vi "arm control.vi"(9 "FPGA_Time_Seconds":dbl format="%33.4f", 10 "appended array":T1[](array[typedef])) -> (2 "appended array 2":dbl[](array[numeric]))   [LabVIEW 2020]
uses:
  <vilib>/Rock Robotics/WPI/MotorControl/WPI_MotorControlDeviceRef.ctl
  <vilib>/Rock Robotics/WPI/MotorControl/WPI_MotorControlType.ctl
  <vilib>/Rock Robotics/SystemInterfaces/DIO/FPGA_DIOPWMChannel.ctl
  <vilib>/Rock Robotics/WPI/PWM/WPI_PWMDeadband.ctl
  <vilib>/Rock Robotics/SystemInterfaces/DIO/FPGA_DIOChannel.ctl
  <vilib>/Rock Robotics/WPI/Joystick/XBox Buttons Indexer.ctl
  <vilib>/Rock Robotics/WPI/Joystick/XBox Axes Indexer.ctl
  <vilib>/Rock Robotics/WPI/ThirdParty/JAS_Junk/TrajLib/PIDController_AtSetpoint.vi
  <vilib>/Rock Robotics/WPI/ThirdParty/JAS_Junk/TrajLib/PIDController_SetPIDF.vi
  <vilib>/Rock Robotics/WPI/ThirdParty/JAS_Junk/TrajLib/PIDController_SetDerivativeFilter.vi
  <vilib>/Rock Robotics/WPI/ThirdParty/JAS_Junk/TrajLib/PIDController_SetIntegratorRange.vi
  <vilib>/Rock Robotics/WPI/ThirdParty/JAS_Junk/TrajLib/PIDController_SetTolerancePandV.vi
  <vilib>/Rock Robotics/WPI/ThirdParty/JAS_Junk/TrajLib/PIDController_DisableContinousInput.vi
  <vilib>/Rock Robotics/WPI/ThirdParty/JAS_Junk/TrajLib/PIDController_EnableContinousInput.vi
  <vilib>/Rock Robotics/WPI/ThirdParty/JAS_Junk/TrajLib/PIDController_Reset.vi
  <vilib>/Rock Robotics/WPI/ThirdParty/JAS_Junk/TrajLib/PIDController_New.vi
  <vilib>/Rock Robotics/WPI/ThirdParty/JAS_Junk/TrajLib/PIDController_SetOutputLimits.vi
  <vilib>/Rock Robotics/WPI/ThirdParty/JAS_Junk/TrajLib/PIDController_NewPeriod.vi
  <vilib>/Rock Robotics/SystemInterfaces/NetworkCommunication/NetComm_UsageReport_report.vi
  Robot Global Data.vi
  <vilib>/Rock Robotics/WPI/ThirdParty/JAS_Junk/TrajLib/Globals/Util_LibraryGlobals.vi
  <vilib>/Rock Robotics/WPI/ThirdParty/JAS_Junk/TrajLib/PIDController_AdvCalculate_FF_Sp_Pv.vi
  <vilib>/Rock Robotics/WPI/ThirdParty/JAS_Junk/TrajLib/Trajectory_Library.lvlib
panel:
  in  "Kp Arm":dbl=0.33 format="%#_13g"
  out "one press\n 5":bool
  out "current angle 5":dbl
  out "current angle 3":dbl
  out "current angle 2":dbl
  out "current angle":dbl
  in  "Kd Grip":dbl format="%#_13g"
  in  "Ki Grip":dbl format="%#_13g"
  in  "Kp Grip":dbl format="%#_13g"
  in  "Kd Wirst":dbl format="%#_13g"
  in  "Ki Wrist":dbl=0.009 format="%#_13g"
  in  "Kp Wrist":dbl=0.06 format="%#_13g"
  in  "Kd Elbow":dbl format="%#_13g"
  in  "Ki Elbow":dbl=0.001 format="%#_13g"
  in  "Kp Elbow":dbl=0.04 format="%#_13g"
  in  "Kd Arm":dbl format="%#_13g"
  in  "Ki Arm":dbl=0.001 format="%#_13g"
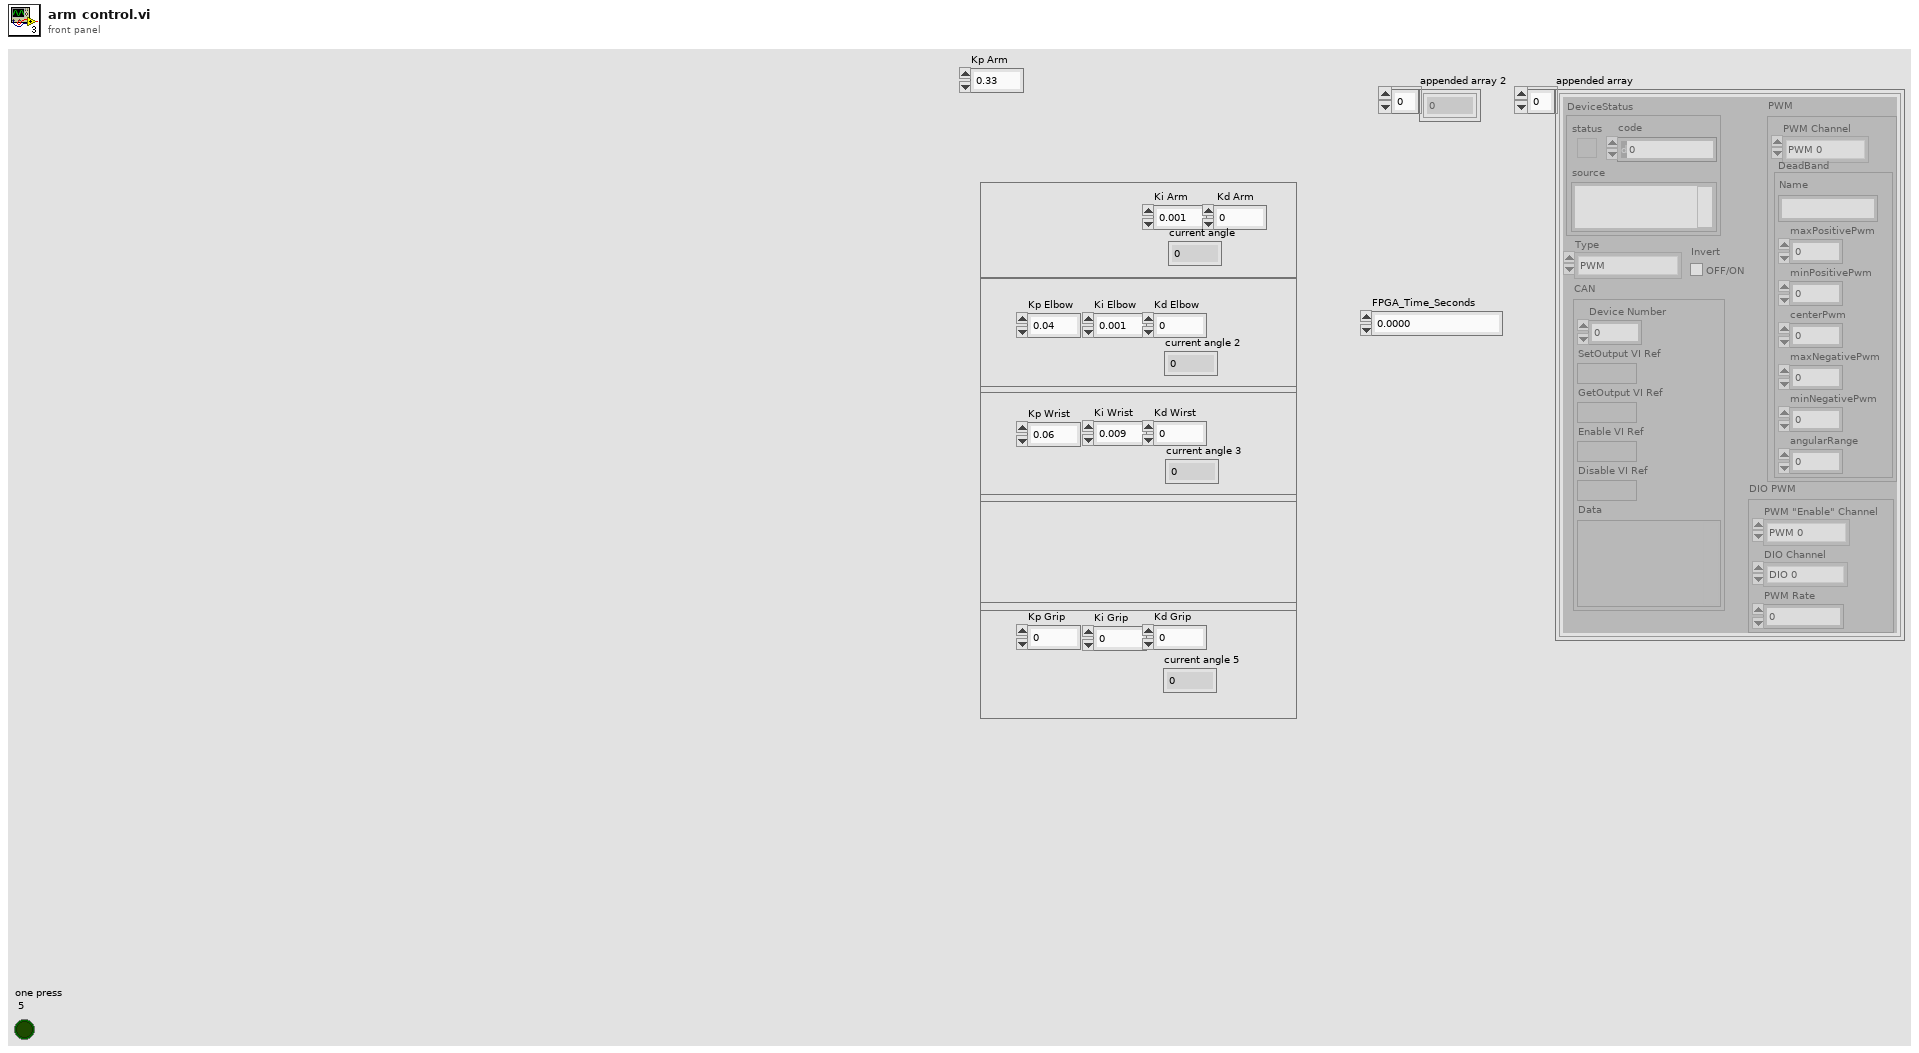
[diagram p1: front panel]
types:
  T1 = typedef "WPI_MotorControlDeviceRef.ctl" = cluster{"DeviceStatus":errorcluster, "Type":T2, "PWM":cluster{"PWM Channel":T3, "DeadBand":T4}, "CAN":cluster{"Device Number":u8, "SetOutput VI Ref":variant, "GetOutput VI Ref":variant, "Enable VI Ref":variant, "Disable VI Ref":variant, "Data":variant}, "Invert":bool, "DIO PWM":cluster{"PWM \"Enable\" Channel":T3, "DIOChannel":T5, "PWM Rate":dbl}}
  T2 = typedef "WPI_MotorControlType.ctl" = enum16{"PWM", "CAN", "DIO PWM"}
  T3 = typedef "FPGA_DIOPWMChannel.ctl" = enum8{"PWM 0", "PWM 1", "PWM 2", "PWM 3", "PWM 4", "PWM 5", "PWM 6", "PWM 7", "PWM 8", "PWM 9", "PWM MXP 0", "PWM MXP 1", "PWM MXP 2", "PWM MXP 3", "PWM MXP 4", "PWM MXP 5", "PWM MXP 6", "PWM MXP 7", "PWM MXP 8", "PWM MXP 9", "Invalid"}
  T4 = typedef "WPI_PWMDeadband.ctl" = cluster{"Name":string, "maxPositivePwm":i32, "minPositivePwm":i32, "centerPwm":i32, "maxNegativePwm":i32, "minNegativePwm":i32, "angularRange":u16}
  T5 = typedef "FPGA_DIOChannel.ctl" = enum8{"DIO 0", "DIO 1", "DIO 2", "DIO 3", "DIO 4", "DIO 5", "DIO 6", "DIO 7", "DIO 8", "DIO 9", "DIO MXP 0", "DIO MXP 1", "DIO MXP 2", "DIO MXP 3", "DIO MXP 4", "DIO MXP 5", "DIO MXP 6", "DIO MXP 7", "DIO MXP 8", "DIO MXP 9", "DIO MXP 10", "DIO MXP 11", "DIO MXP 12", "DIO MXP 13", "DIO MXP 14", "DIO MXP 15", "SPI Port CS1", "SPI Port CS2", "SPI Port CS3", "SPI Port MISO", "SPI Port MOSI", "Invalid"}
  T6 = typedef "XBox Buttons Indexer.ctl" = enum16{"A", "B", "X", "Y", "Left Bumper", "Right Bumper", "Back", "Start", "Left Joystick", "Right Joystick"}
  T7 = typedef "XBox Axes Indexer.ctl" = enum16{"Left X", "Left Y", "Left Trigger", "Right Trigger", "Right X", "Right Y"}
  T8 = typedef "Trajectory_Library.lvlib/PID_ADV_LIMITS.ctl" = cluster{"MaxInput":dbl, "MinInput":dbl, "Continuous":bool, "MaxOutput":dbl, "MinOutput":dbl}
  T9 = typedef "Trajectory_Library.lvlib/PID_ADV_TUNING.ctl" = cluster{"Kf":dbl, "Kp":dbl, "Ki":dbl, "Kd":dbl, "MaximumIntegral":dbl, "MinimumIntegral":dbl, "Filter Derivative":bool}
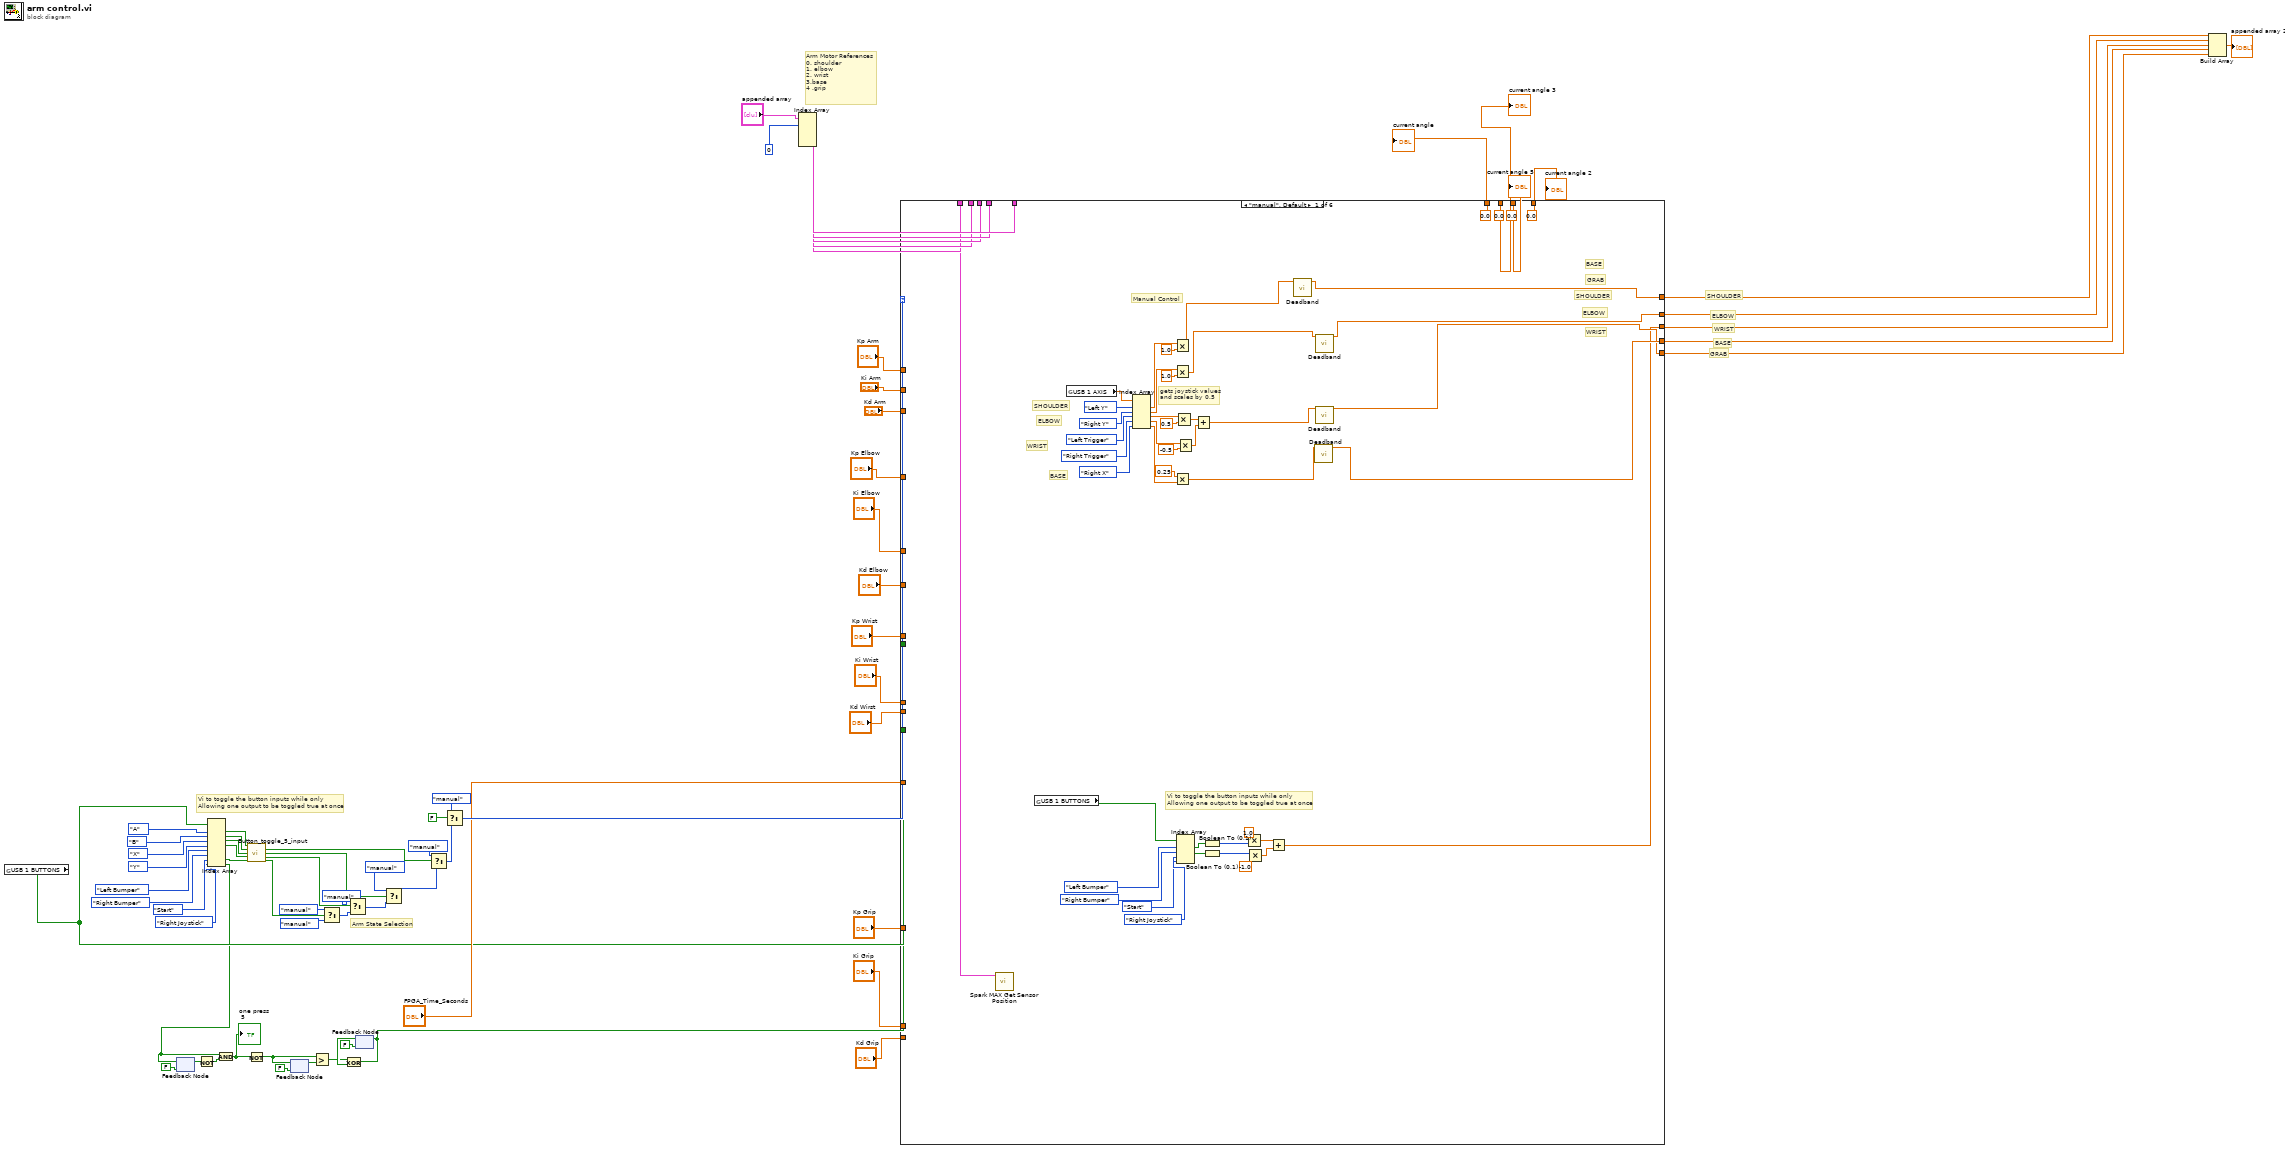
[diagram p0: block diagram]
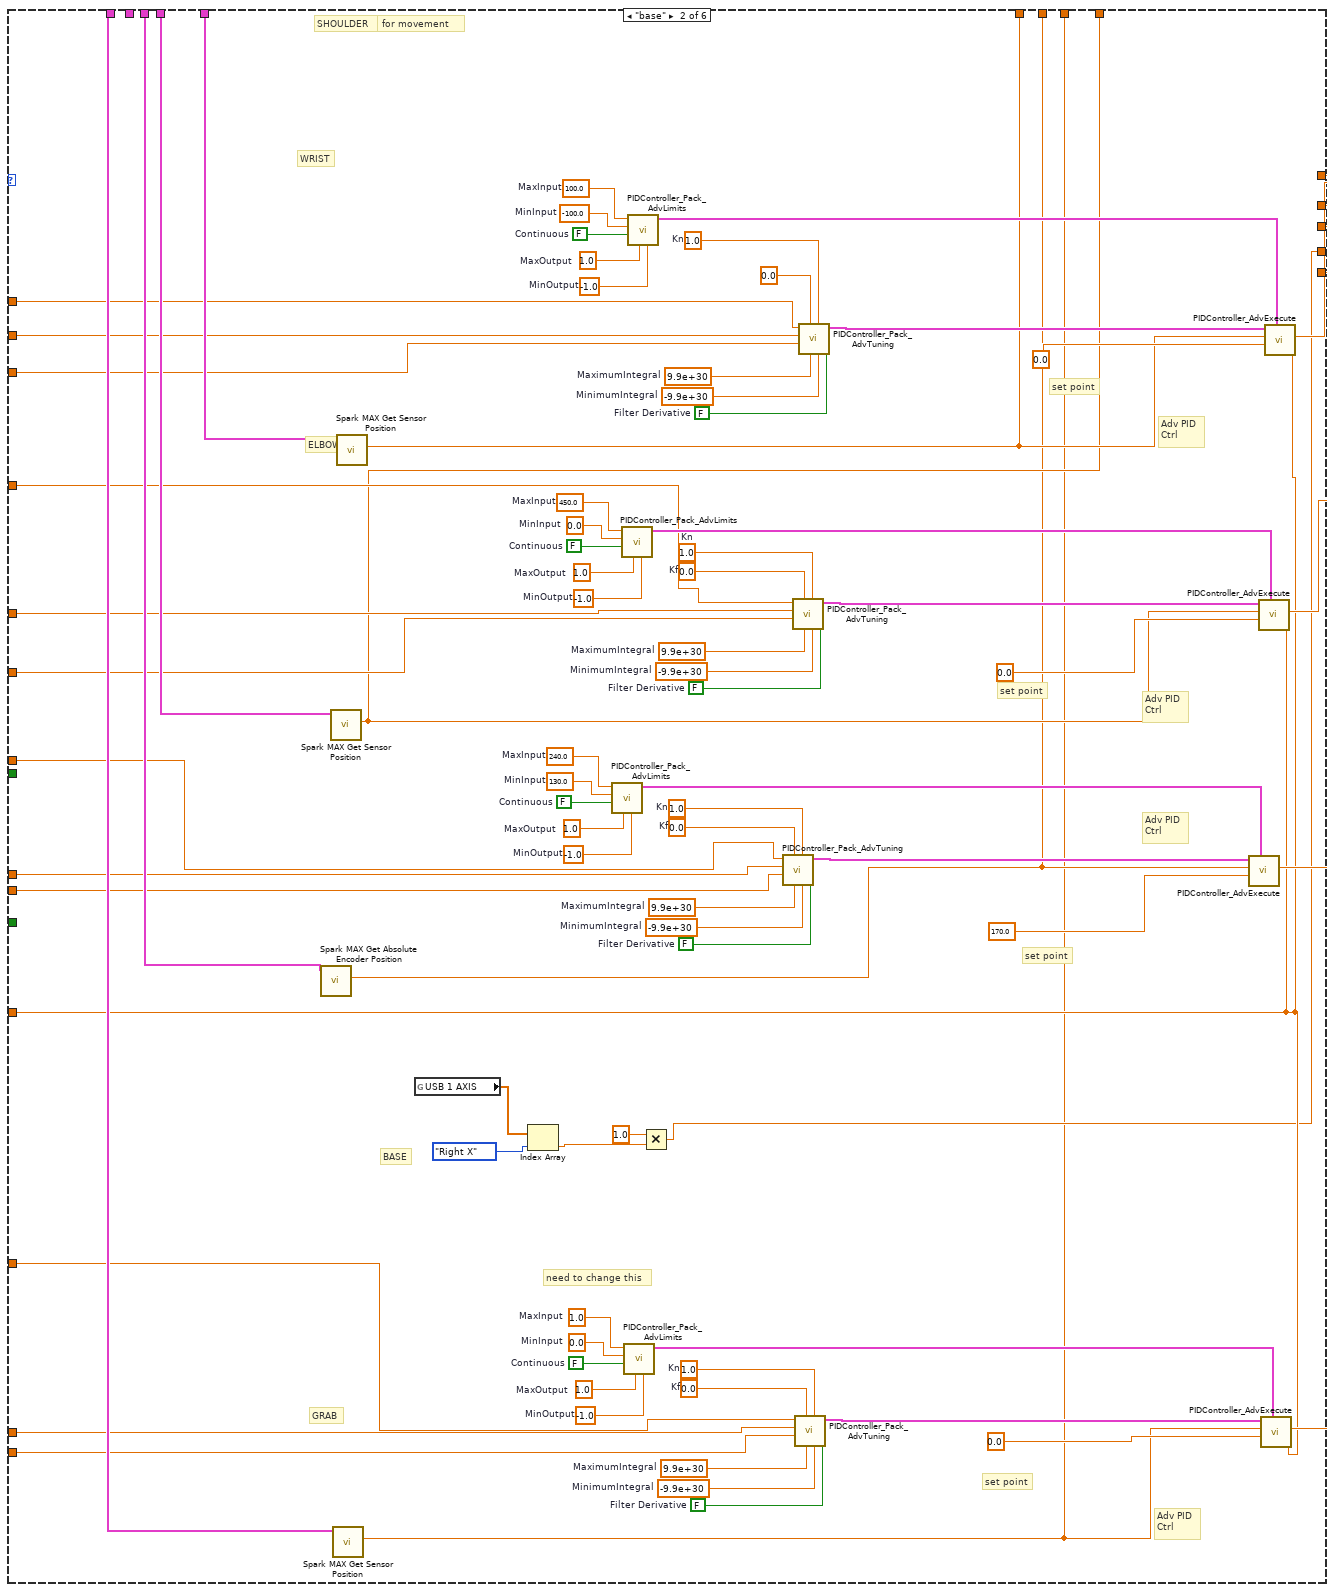
[diagram p2: hidden frame]
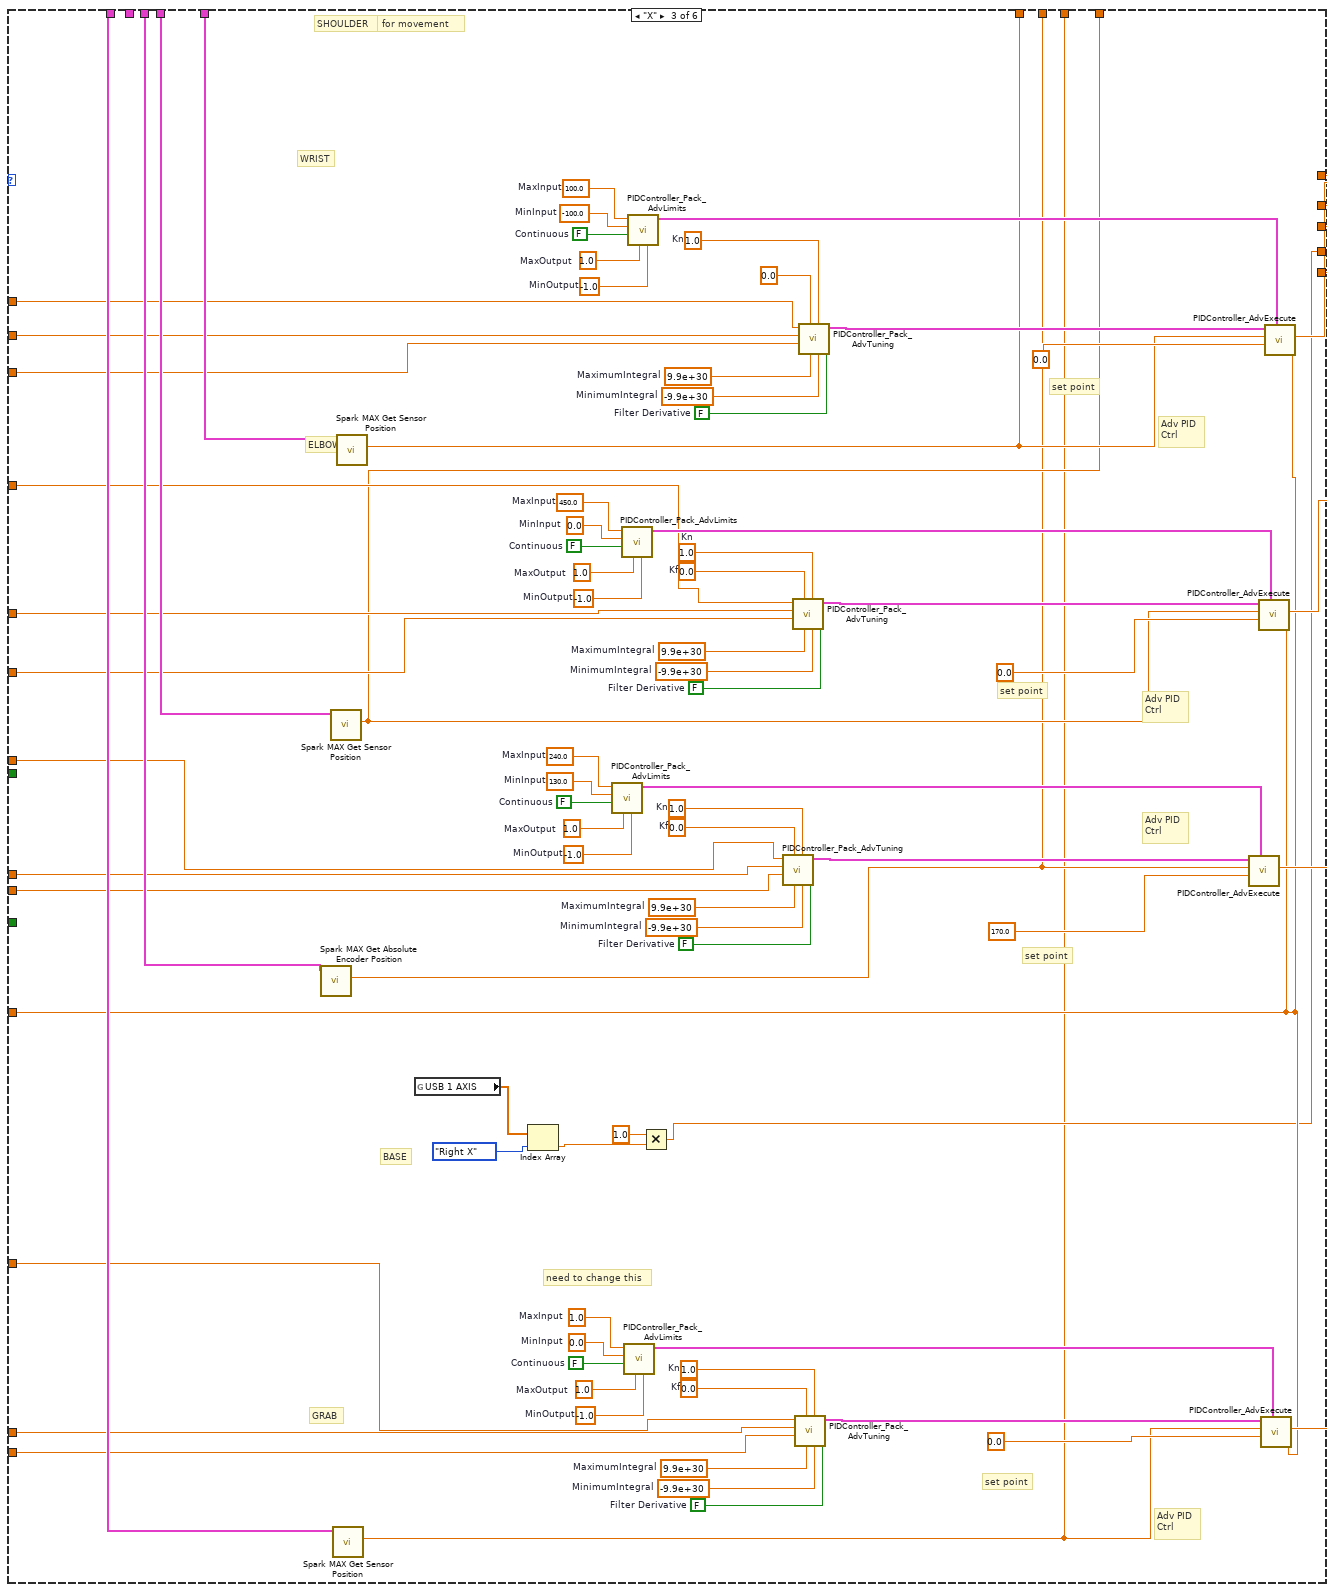
[diagram p3: hidden frame]
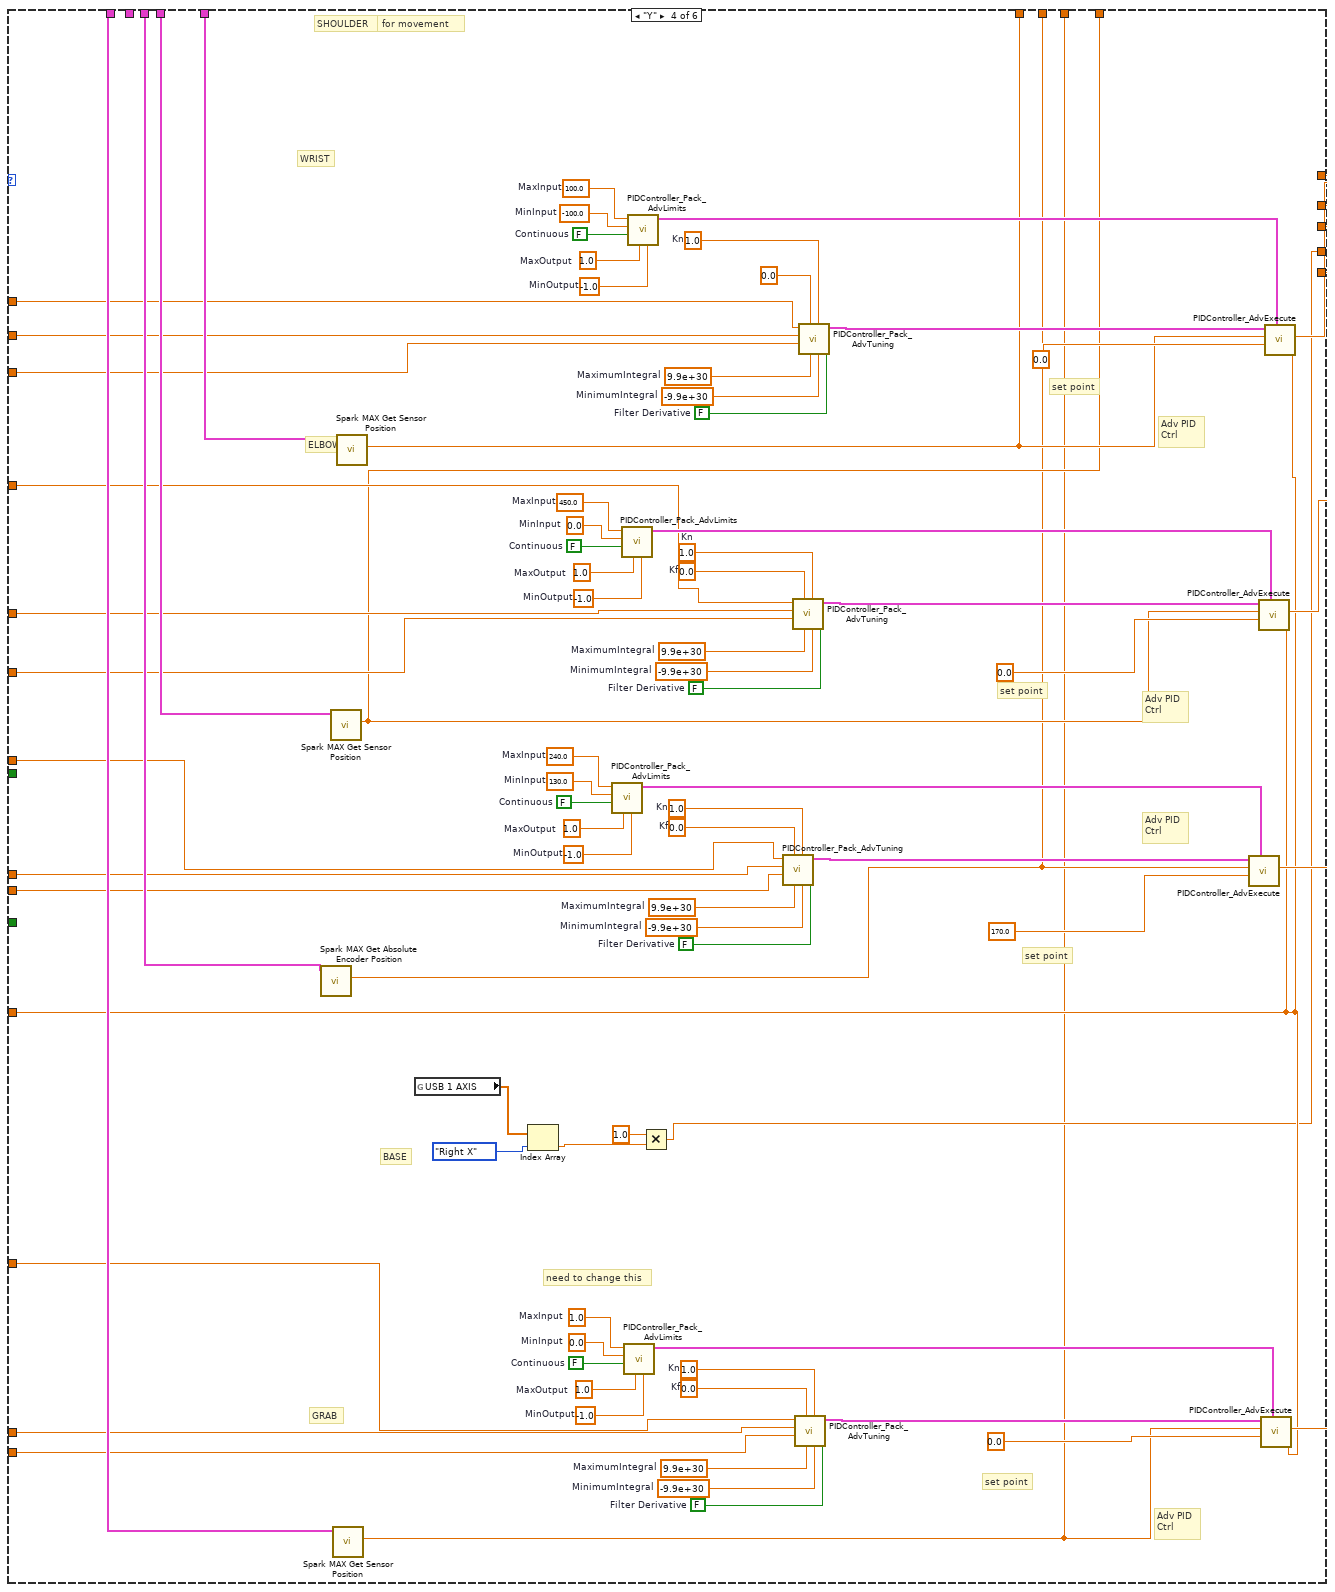
[diagram p4: hidden frame]
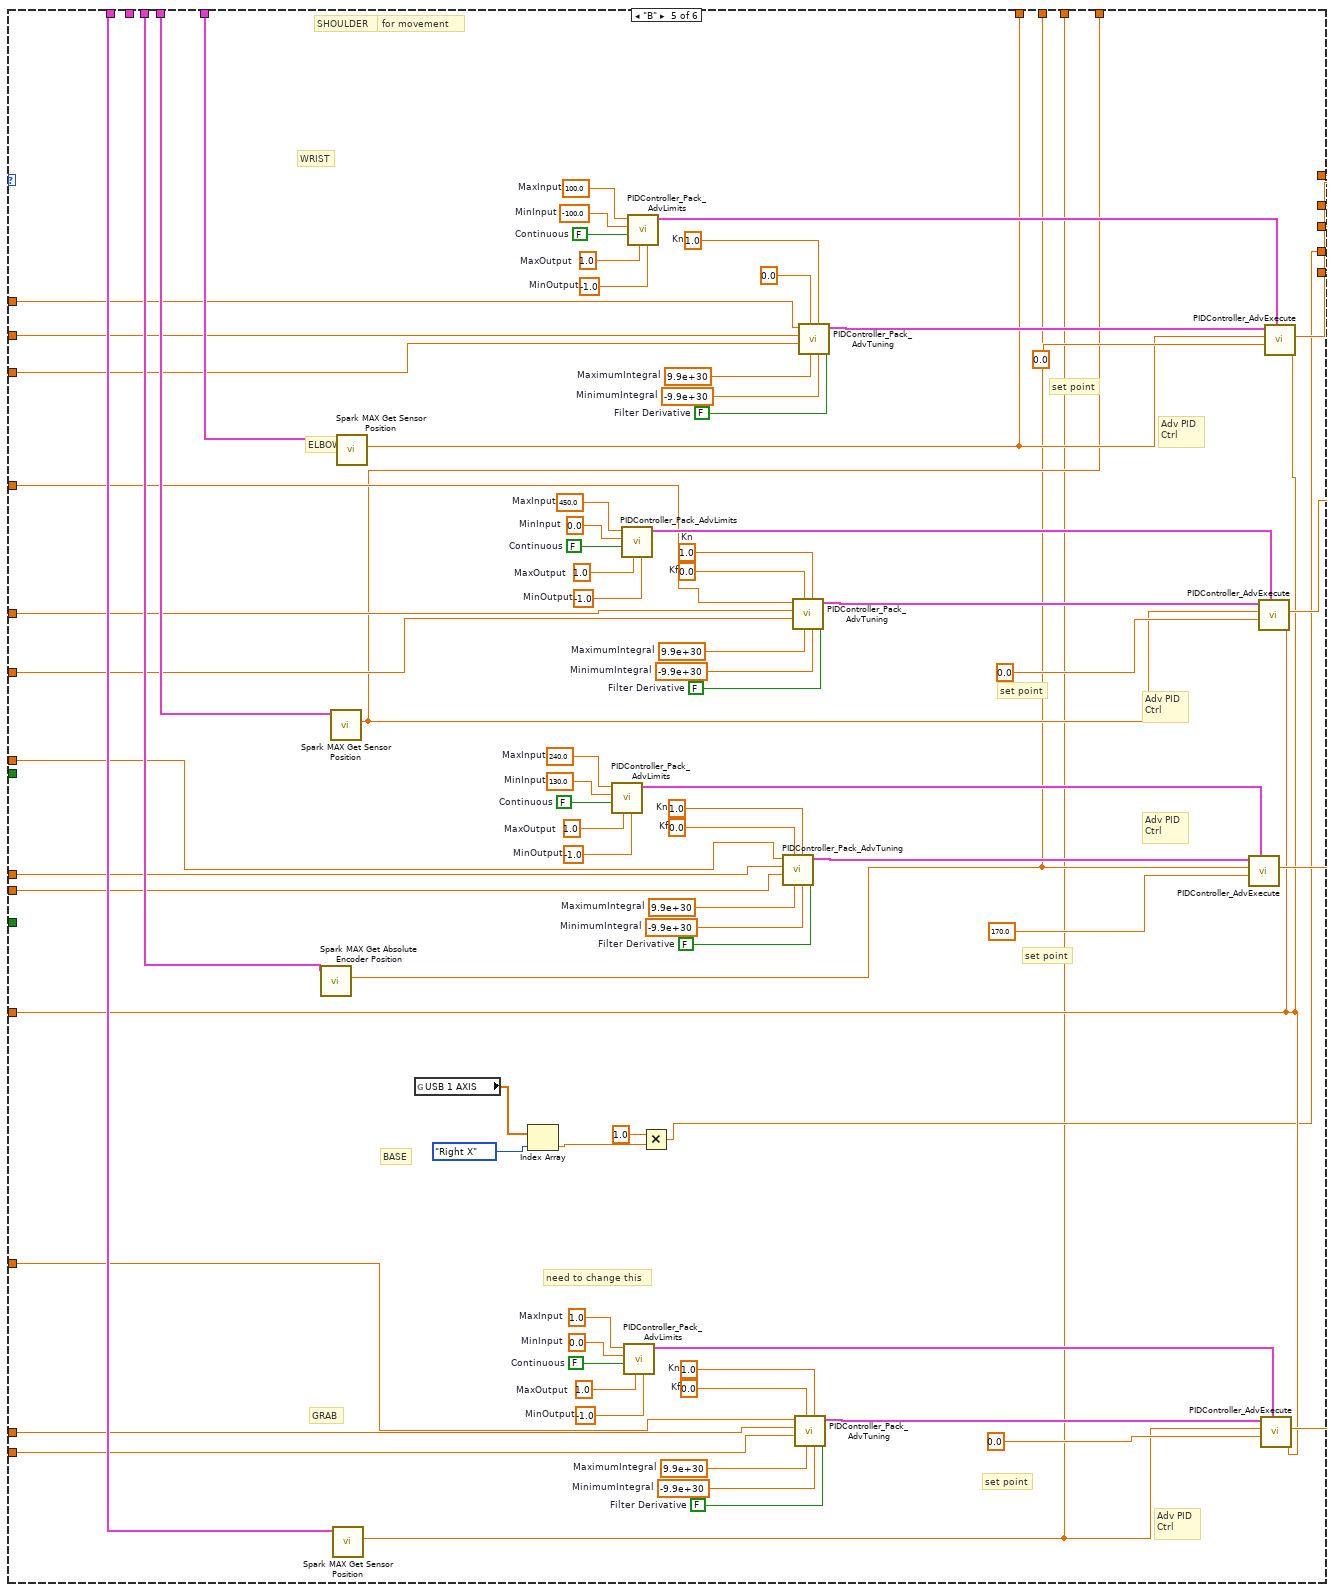
[diagram p5: hidden frame]
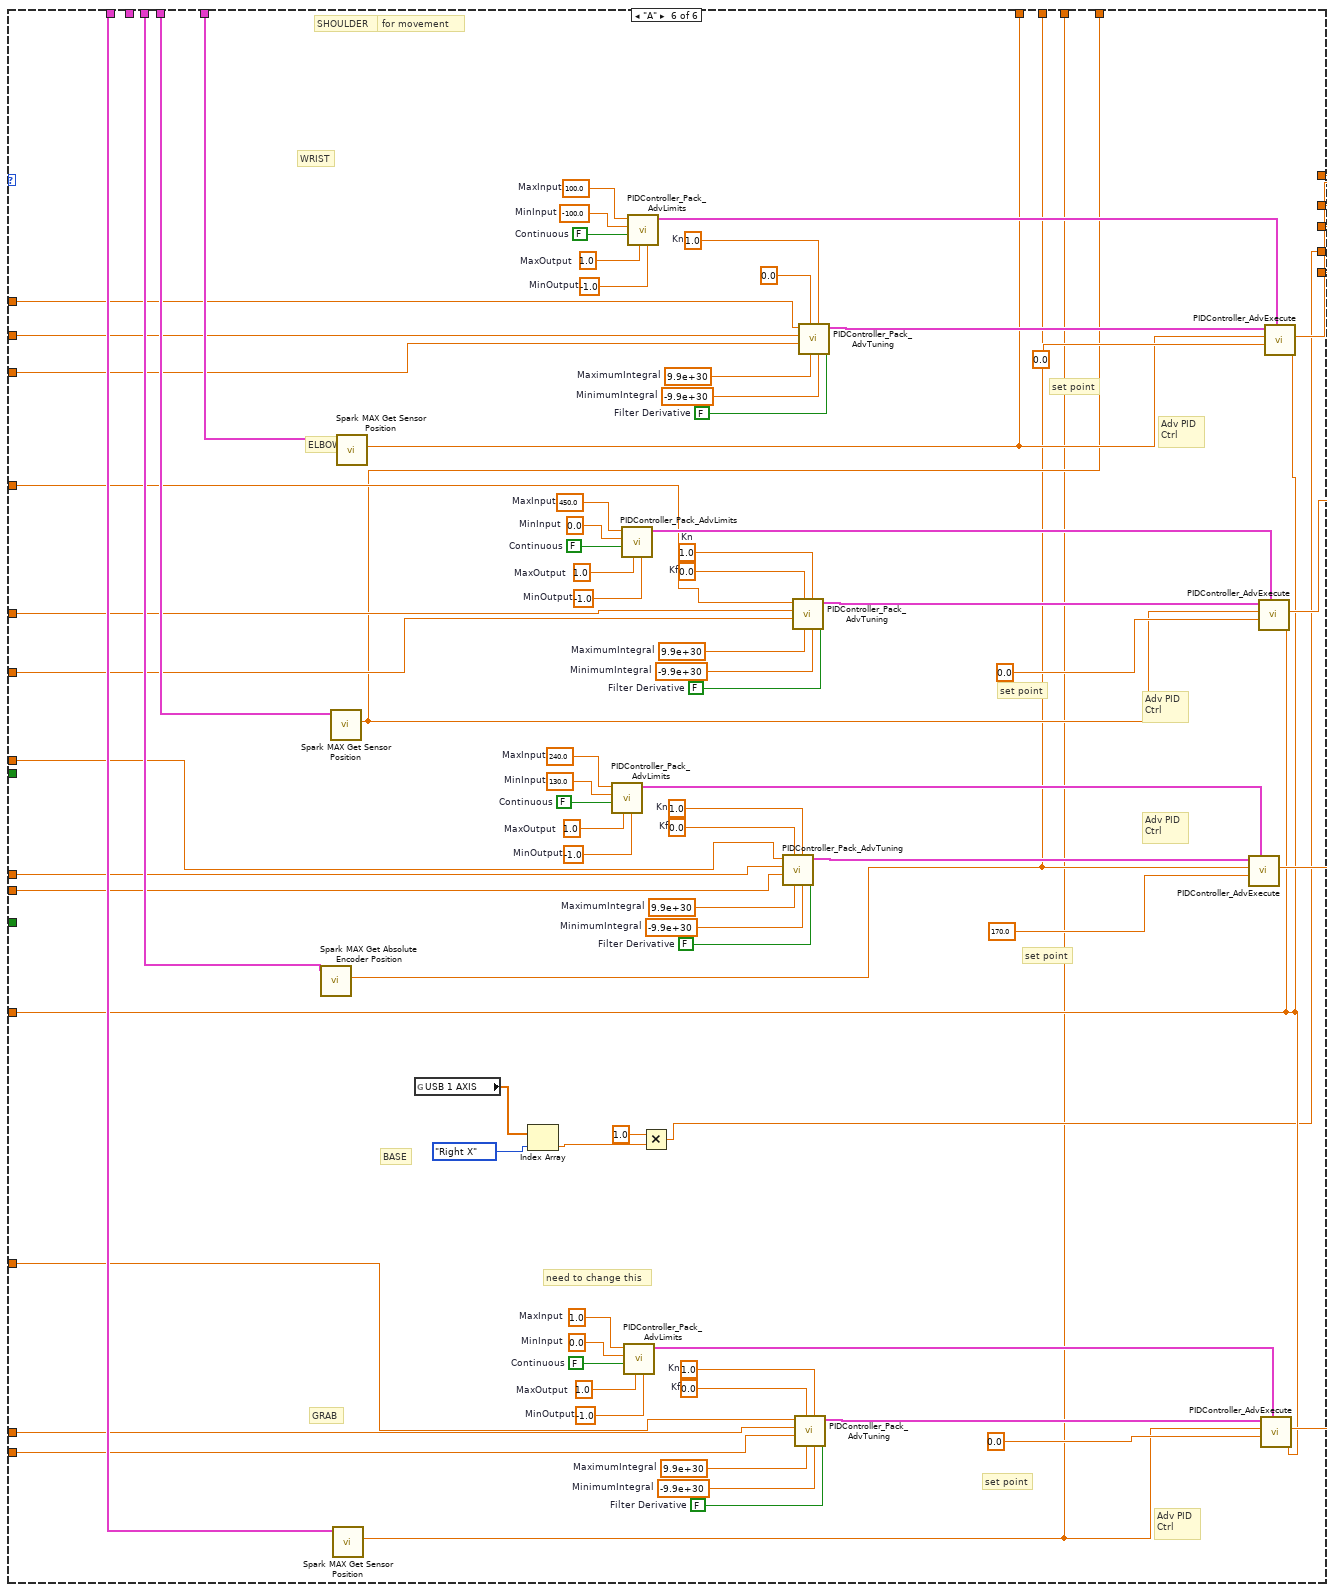
[diagram p6: hidden frame]
diagram:
  # "Arm Motor References\n0. shoulder\n1. elbow\n2. wrist\n3.base\n4 .grip"
  # "Arm State Selection"
  # "Vi to toggle the button inputs while only \nAllowing one output to be toggled true at once"
  # "GRAB"
  # "BASE"
  # "WRIST"
  # "ELBOW"
  # "SHOULDER"
  n1 = global read "Robot Global Data.vi" "USB 1 BUTTONS"() -> (w31:bool[])
  n2 = feedback #1(FALSE) -> (w26:bool)
  n3 = Not(x=w26) -> (.not. x?=w27:bool)
  n4 = Index Array(array=w31, index #1=XBox_Buttons_Indexer."A" ("XBox Buttons"), index #2=XBox_Buttons_Indexer."B" ("XBox Buttons"), index #3=XBox_Buttons_Indexer."X" ("XBox Buttons"), index #4=XBox_Buttons_Indexer."Y" ("XBox Buttons"), index #5=XBox_Buttons_Indexer."Left Bumper" ("XBox Buttons"), index #6=XBox_Buttons_Indexer."Right Bumper" ("XBox Buttons"), index #7=XBox_Buttons_Indexer."Start" ("XBox Buttons"), index #8=XBox_Buttons_Indexer."Right Joystick" ("XBox Buttons")) -> (element #1=w64:bool, element #2=w65:bool, element #3=w66:bool, element #4=w67:bool, element #7=w68:bool, element #8=w17:bool)  [unwired: 2 out]
  n5 = feedback-in #1(w17) -> ()
  n6 = And(x=w17, y=w27) -> (x .and. y?=w25:bool)
  "one press\n 5" <- w25
  n7 = call "Button_toggle_5_input.vi"("in 1"=w64, "in 2"=w65, "in3"=w66, "in 4"=w67, "in 5"=w68) -> ("Out 2"=w69:bool, "Out3"=w70:bool, "Out 4"=w71:bool, "out 5"=w72:bool)  [unwired: 6 in, 1 out]
  n8 = Not(x=w25) -> (.not. x?=w20:bool)
  n9 = feedback #2(FALSE) -> (w21:bool)
  n10 = feedback-in #2(w20) -> ()
  n11 = Greater?(x=w20, y=w21) -> (0:w19:bool)
  n12 = Select(t=enum16{"A", "B", "base", "manual", "X", "Y"}."manual", s=w72, f=enum16{"A", "B", "base", "manual", "X", "Y"}."manual") -> (s? t:f=w56:enum16{"A", "B", "base", "manual", "X", "Y"})
  n13 = Select(t=enum16{"A", "B", "base", "manual", "X", "Y"}."manual", s=w71, f=w56) -> (s? t:f=w54:enum16{"A", "B", "base", "manual", "X", "Y"})
  n14 = feedback #3(FALSE) -> (w22:bool)
  n15 = Exclusive Or(1:w22, 2:w19) -> (0:w18:bool)
  n16 = feedback-in #3(w18) -> ()
  n17 = Select(t=enum16{"A", "B", "base", "manual", "X", "Y"}."manual", s=w70, f=w54) -> (s? t:f=w53:enum16{"A", "B", "base", "manual", "X", "Y"})
  n18 = Select(t=enum16{"A", "B", "base", "manual", "X", "Y"}."manual", s=w69, f=w53) -> (s? t:f=w52:enum16{"A", "B", "base", "manual", "X", "Y"})
  n19 = Select(t=enum16{"A", "B", "base", "manual", "X", "Y"}."manual", s=FALSE, f=w52) -> (s? t:f=w55:enum16{"A", "B", "base", "manual", "X", "Y"})
  n20 = Index Array(array="appended array", index #1=0 ("index")) -> (element #1=w43:T1, element #2=w42:T1, element #3=w41:T1, element #4=w40:T1, element #5=w39:T1)  [unwired: 4 in]
  n21 = case shown="\"manual\", Default" w55 {
    tunnel: [w93 w185 w267 w349 w431 w513] -> w38
    tunnel: [w91 w170 w252 w334 w416 w498] -> w37
    tunnel: [w73 w155 w237 w319 w401 w483] -> w36
    tunnel: [w88 w134 w216 w298 w380 w462] -> w35
    tunnel: [w82 w140 w222 w304 w386 w468] -> w34
    tunnel: w43 -> [_ w186 w268 w350 w432 w514]
    tunnel: w42 -> [_ w171 w253 w335 w417 w499]
    tunnel: w41 -> [_ w156 w238 w320 w402 w484]
    tunnel: w40 -> [_ _ _ _ _ _]
    tunnel: w39 -> [w99 w141 w223 w305 w387 w469]
    tunnel: "FPGA_Time_Seconds" -> [_ w139 w221 w303 w385 w467]
    tunnel: w31 -> [_ _ _ _ _ _]
    tunnel: w18 -> [_ _ _ _ _ _]
    tunnel: "Kp Arm" -> [_ w133 w215 w297 w379 w461]
    tunnel: "Ki Arm" -> [_ w132 w214 w296 w378 w460]
    tunnel: "Kd Arm" -> [_ w131 w213 w295 w377 w459]
    tunnel: "Kp Elbow" -> [_ w130 w212 w294 w376 w458]
    tunnel: "Ki Elbow" -> [_ w129 w211 w293 w375 w457]
    tunnel: "Kd Elbow" -> [_ w128 w210 w292 w374 w456]
    tunnel: "Kd Wirst" -> [_ w127 w209 w291 w373 w455]
    tunnel: "Kp Wrist" -> [_ w126 w208 w290 w372 w454]
    tunnel: "Ki Wrist" -> [_ w125 w207 w289 w371 w453]
    tunnel: "Ki Grip" -> [_ w124 w206 w288 w370 w452]
    tunnel: "Kp Grip" -> [_ w123 w205 w287 w369 w451]
    tunnel: "Kd Grip" -> [_ w122 w204 w286 w368 w450]
    tunnel: [0.0 ("Sensor Position") w121 w203 w285 w367 w449] -> w4
    tunnel: [0.0 ("Sensor Position") w120 w202 w284 w366 w448] -> w3
    tunnel: [0.0 ("Position") w119 w201 w283 w365 w447] -> w2
    tunnel: [0.0 ("Sensor Position") w118 w200 w282 w364 w446] -> w1
    frame "manual", Default {
      # "Vi to toggle the button inputs while only \nAllowing one output to be toggled true at once"
      # "BASE"
      # "WRIST"
      # "ELBOW"
      # "SHOULDER"
      # "gets joystick values\nand scales by 0.5"
      # "Manual Control"
      # "GRAB"
      # "BASE"
      # "WRIST"
      # "ELBOW"
      # "SHOULDER"
      n22 = call <vilib>:"Spark MAX Get Sensor Position.vi"("MotorControlDevRef in"=w99) -> ()  [unwired: 7 in, 4 out]
      n23 = global read "Robot Global Data.vi" "USB 1 BUTTONS"() -> (w86:bool[])
      n24 = global read "Robot Global Data.vi" "USB 1 AXIS"() -> (w103:dbl[])
      n25 = Index Array(array=w103, index #1=XBox_Axes_Indexer."Left Y" ("XBox Axes"), index #2=XBox_Axes_Indexer."Right Y" ("XBox Axes"), index #3=XBox_Axes_Indexer."Left Trigger" ("XBox Axes"), index #4=XBox_Axes_Indexer."Right Trigger" ("XBox Axes"), index #5=XBox_Axes_Indexer."Right X" ("XBox Axes")) -> (element #1=w113:dbl, element #2=w112:dbl, element #3=w111:dbl, element #4=w110:dbl, element #5=w101:dbl)
      n26 = Multiply(x=w113, y=1.0) -> (x*y=w94:dbl)
      n27 = Multiply(x=w112, y=1.0) -> (x*y=w92:dbl)
      n28 = Multiply(x=0.25, y=w101) -> (x*y=w89:dbl)
      n29 = Multiply(x=w111, y=0.5) -> (x*y=w105:dbl)
      n30 = Index Array(array=w86, index #1=XBox_Buttons_Indexer."Left Bumper" ("XBox Buttons"), index #2=XBox_Buttons_Indexer."Right Bumper" ("XBox Buttons"), index #3=XBox_Buttons_Indexer."Start" ("XBox Buttons"), index #4=XBox_Buttons_Indexer."Right Joystick" ("XBox Buttons")) -> (element #1=w77:bool, element #2=w76:bool)  [unwired: 2 out]
      n31 = Multiply(x=w110, y=-0.5) -> (x*y=w104:dbl)
      n32 = Add(x=w105, y=w104) -> (x+y=w90:dbl)
      n33 = Boolean To (0,1)(Boolean=w77) -> (0, 1=w75:i16)
      n34 = Boolean To (0,1)(Boolean=w76) -> (0, 1=w74:i16)
      n35 = Multiply(x=1.0, y=w75) -> (x*y=w81:dbl)
      n36 = Multiply(x=w74, y=-1.0) -> (x*y=w80:dbl)
      n37 = Add(x=w81, y=w80) -> (x+y=w73:dbl)
      n38 = call "Deadband.vi"("upper limit"=w94) -> ("Numeric"=w93:dbl)  [unwired: 9 in, 1 out]
      n39 = call "Deadband.vi"("upper limit"=w89) -> ("Numeric"=w88:dbl)  [unwired: 9 in, 1 out]
      n40 = call "Deadband.vi"("upper limit"=w92) -> ("Numeric"=w91:dbl)  [unwired: 9 in, 1 out]
      n41 = call "Deadband.vi"("upper limit"=w90) -> ("Numeric"=w82:dbl)  [unwired: 9 in, 1 out]
    }
    frame "base" {
      w154 = 1.0  # Kn
      w153 = 0.0  # Kf
      w143 = 9.9e+30  # MaximumIntegral
      w152 = -9.9e+30  # MinimumIntegral
      w151 = FALSE  # Filter Derivative
      w149 = 0.0  # MinInput
      w148 = FALSE  # Continuous
      w147 = 1.0  # MaxOutput
      w150 = -1.0  # MinOutput
      w146 = 1.0  # MaxInput
      w169 = 1.0  # Kn
      w168 = 0.0  # Kf
      w158 = 9.9e+30  # MaximumIntegral
      w167 = -9.9e+30  # MinimumIntegral
      w166 = FALSE  # Filter Derivative
      w164 = 130.0  # MinInput
      w163 = FALSE  # Continuous
      w162 = 1.0  # MaxOutput
      w165 = -1.0  # MinOutput
      w161 = 240.0  # MaxInput
      w184 = 1.0  # Kn
      w183 = 0.0  # Kf
      w173 = 9.9e+30  # MaximumIntegral
      w182 = -9.9e+30  # MinimumIntegral
      w181 = FALSE  # Filter Derivative
      w179 = 0.0  # MinInput
      w178 = FALSE  # Continuous
      w177 = 1.0  # MaxOutput
      w180 = -1.0  # MinOutput
      w176 = 450.0  # MaxInput
      w187 = 1.0  # Kn
      w198 = 9.9e+30  # MaximumIntegral
      w189 = -9.9e+30  # MinimumIntegral
      w190 = FALSE  # Filter Derivative
      w192 = -100.0  # MinInput
      w193 = FALSE  # Continuous
      w194 = 1.0  # MaxOutput
      w191 = -1.0  # MinOutput
      w195 = 100.0  # MaxInput
      # "set point"
      # "BASE"
      # "set point"
      # "set point"
      # "set point"
      # "base postion for movement"
      # "GRAB"
      # "WRIST"
      # "ELBOW"
      # "SHOULDER"
      # "need to change this"
      # "Adv PID\nCtrl"
      # "Adv PID\nCtrl"
      # "Adv PID\nCtrl"
      # "Adv PID\nCtrl"
      n42 = call <vilib>:"Spark MAX Get Absolute Encoder Position.vi"("MotorControlDeviceRef in"=w156) -> ("Position"=w119:dbl)  [unwired: 7 in, 3 out]
      n43 = call <vilib>:"Spark MAX Get Sensor Position.vi"("MotorControlDevRef in"=w171) -> ("Sensor Position"=w120:dbl)  [unwired: 7 in, 3 out]
      n44 = call <vilib>:"Spark MAX Get Sensor Position.vi"("MotorControlDevRef in"=w141) -> ("Sensor Position"=w118:dbl)  [unwired: 7 in, 3 out]
      n45 = call <vilib>:"Spark MAX Get Sensor Position.vi"("MotorControlDevRef in"=w186) -> ("Sensor Position"=w121:dbl)  [unwired: 7 in, 3 out]
      n46 = global read "Robot Global Data.vi" "USB 1 AXIS"() -> (w138:dbl[])
      n47 = Index Array(array=w138, index=XBox_Axes_Indexer."Right X" ("XBox Axes")) -> (element=w136:dbl)
      n48 = call <vilib>:"PIDController_Pack_AdvLimits.vi"("MinOutput"=w165, "MaxOutput"=w162, "Continuous"=w163, "MinInput"=w164, "MaxInput"=w161) -> ("Adv PID Limits"=w159:T8)  [unwired: 6 in]
      n49 = call <vilib>:"PIDController_Pack_AdvLimits.vi"("MinOutput"=w180, "MaxOutput"=w177, "Continuous"=w178, "MinInput"=w179, "MaxInput"=w176) -> ("Adv PID Limits"=w174:T8)  [unwired: 6 in]
      n50 = call <vilib>:"PIDController_Pack_AdvLimits.vi"("MinOutput"=w150, "MaxOutput"=w147, "Continuous"=w148, "MinInput"=w149, "MaxInput"=w146) -> ("Adv PID Limits"=w144:T8)  [unwired: 6 in]
      n51 = call <vilib>:"PIDController_Pack_AdvLimits.vi"("MinOutput"=w191, "MaxOutput"=w194, "Continuous"=w193, "MinInput"=w192, "MaxInput"=w195) -> ("Adv PID Limits"=w197:T8)  [unwired: 6 in]
      n52 = Multiply(x=1.0, y=w136) -> (x*y=w134:dbl)
      n53 = call <vilib>:"PIDController_Pack_AdvTuning.vi"("Filter Derivative"=w166, "MinimumIntegral"=w167, "Kn"=w169, "MaximumIntegral"=w158, "Kf"=w168, "Kd"=w127, "Ki"=w125, "Kp"=w126) -> ("Adv PID Tuning"=w160:T9)  [unwired: 3 in]
      n54 = call <vilib>:"PIDController_Pack_AdvTuning.vi"("Filter Derivative"=w181, "MinimumIntegral"=w182, "Kn"=w184, "MaximumIntegral"=w173, "Kf"=w183, "Kd"=w128, "Ki"=w129, "Kp"=w130) -> ("Adv PID Tuning"=w175:T9)  [unwired: 3 in]
      n55 = call <vilib>:"PIDController_Pack_AdvTuning.vi"("Filter Derivative"=w151, "MinimumIntegral"=w152, "Kn"=w154, "MaximumIntegral"=w143, "Kf"=w153, "Kd"=w122, "Ki"=w124, "Kp"=w123) -> ("Adv PID Tuning"=w145:T9)  [unwired: 3 in]
      n56 = call <vilib>:"PIDController_Pack_AdvTuning.vi"("Filter Derivative"=w190, "MinimumIntegral"=w189, "Kn"=w187, "MaximumIntegral"=w198, "Kf"=0.0 ("Kf Arm"), "Kd"=w131, "Ki"=w132, "Kp"=w133) -> ("Adv PID Tuning"=w196:T9)  [unwired: 3 in]
      n57 = call <vilib>:"PIDController_AdvExecute.vi"("Adv PID Limits"=w159, "SP-SetPoint"=170.0 ("Wrist Setpoint"), "PV-Measurement"=w119, "Adv PID Tuning"=w160) -> ("CO-ControlOutput"=w155:dbl)  [unwired: 5 in, 2 out]
      n58 = call <vilib>:"PIDController_AdvExecute.vi"("Time"=w139, "Adv PID Limits"=w174, "SP-SetPoint"=0.0 ("Setpoit Elbow"), "PV-Measurement"=w120, "Adv PID Tuning"=w175) -> ("CO-ControlOutput"=w170:dbl)  [unwired: 4 in, 2 out]
      n59 = call <vilib>:"PIDController_AdvExecute.vi"("Time"=w139, "Adv PID Limits"=w144, "SP-SetPoint"=0.0 ("set point grip"), "PV-Measurement"=w118, "Adv PID Tuning"=w145) -> ("CO-ControlOutput"=w140:dbl)  [unwired: 4 in, 2 out]
      n60 = call <vilib>:"PIDController_AdvExecute.vi"("Time"=w139, "Adv PID Limits"=w197, "SP-SetPoint"=0.0 ("set poit arm"), "PV-Measurement"=w121, "Adv PID Tuning"=w196) -> ("CO-ControlOutput"=w185:dbl)  [unwired: 4 in, 2 out]
    }
    frame "X" {
      w236 = 1.0  # Kn
      w235 = 0.0  # Kf
      w225 = 9.9e+30  # MaximumIntegral
      w234 = -9.9e+30  # MinimumIntegral
      w233 = FALSE  # Filter Derivative
      w231 = 0.0  # MinInput
      w230 = FALSE  # Continuous
      w229 = 1.0  # MaxOutput
      w232 = -1.0  # MinOutput
      w228 = 1.0  # MaxInput
      w251 = 1.0  # Kn
      w250 = 0.0  # Kf
      w240 = 9.9e+30  # MaximumIntegral
      w249 = -9.9e+30  # MinimumIntegral
      w248 = FALSE  # Filter Derivative
      w246 = 130.0  # MinInput
      w245 = FALSE  # Continuous
      w244 = 1.0  # MaxOutput
      w247 = -1.0  # MinOutput
      w243 = 240.0  # MaxInput
      w266 = 1.0  # Kn
      w265 = 0.0  # Kf
      w255 = 9.9e+30  # MaximumIntegral
      w264 = -9.9e+30  # MinimumIntegral
      w263 = FALSE  # Filter Derivative
      w261 = 0.0  # MinInput
      w260 = FALSE  # Continuous
      w259 = 1.0  # MaxOutput
      w262 = -1.0  # MinOutput
      w258 = 450.0  # MaxInput
      w269 = 1.0  # Kn
      w280 = 9.9e+30  # MaximumIntegral
      w271 = -9.9e+30  # MinimumIntegral
      w272 = FALSE  # Filter Derivative
      w274 = -100.0  # MinInput
      w275 = FALSE  # Continuous
      w276 = 1.0  # MaxOutput
      w273 = -1.0  # MinOutput
      w277 = 100.0  # MaxInput
      # "set point"
      # "BASE"
      # "set point"
      # "set point"
      # "set point"
      # "base postion for movement"
      # "GRAB"
      # "WRIST"
      # "ELBOW"
      # "SHOULDER"
      # "need to change this"
      # "Adv PID\nCtrl"
      # "Adv PID\nCtrl"
      # "Adv PID\nCtrl"
      # "Adv PID\nCtrl"
      n61 = call <vilib>:"Spark MAX Get Absolute Encoder Position.vi"("MotorControlDeviceRef in"=w238) -> ("Position"=w201:dbl)  [unwired: 7 in, 3 out]
      n62 = call <vilib>:"Spark MAX Get Sensor Position.vi"("MotorControlDevRef in"=w253) -> ("Sensor Position"=w202:dbl)  [unwired: 7 in, 3 out]
      n63 = call <vilib>:"Spark MAX Get Sensor Position.vi"("MotorControlDevRef in"=w223) -> ("Sensor Position"=w200:dbl)  [unwired: 7 in, 3 out]
      n64 = call <vilib>:"Spark MAX Get Sensor Position.vi"("MotorControlDevRef in"=w268) -> ("Sensor Position"=w203:dbl)  [unwired: 7 in, 3 out]
      n65 = global read "Robot Global Data.vi" "USB 1 AXIS"() -> (w220:dbl[])
      n66 = Index Array(array=w220, index=XBox_Axes_Indexer."Right X" ("XBox Axes")) -> (element=w218:dbl)
      n67 = call <vilib>:"PIDController_Pack_AdvLimits.vi"("MinOutput"=w247, "MaxOutput"=w244, "Continuous"=w245, "MinInput"=w246, "MaxInput"=w243) -> ("Adv PID Limits"=w241:T8)  [unwired: 6 in]
      n68 = call <vilib>:"PIDController_Pack_AdvLimits.vi"("MinOutput"=w262, "MaxOutput"=w259, "Continuous"=w260, "MinInput"=w261, "MaxInput"=w258) -> ("Adv PID Limits"=w256:T8)  [unwired: 6 in]
      n69 = call <vilib>:"PIDController_Pack_AdvLimits.vi"("MinOutput"=w232, "MaxOutput"=w229, "Continuous"=w230, "MinInput"=w231, "MaxInput"=w228) -> ("Adv PID Limits"=w226:T8)  [unwired: 6 in]
      n70 = call <vilib>:"PIDController_Pack_AdvLimits.vi"("MinOutput"=w273, "MaxOutput"=w276, "Continuous"=w275, "MinInput"=w274, "MaxInput"=w277) -> ("Adv PID Limits"=w279:T8)  [unwired: 6 in]
      n71 = Multiply(x=1.0, y=w218) -> (x*y=w216:dbl)
      n72 = call <vilib>:"PIDController_Pack_AdvTuning.vi"("Filter Derivative"=w248, "MinimumIntegral"=w249, "Kn"=w251, "MaximumIntegral"=w240, "Kf"=w250, "Kd"=w209, "Ki"=w207, "Kp"=w208) -> ("Adv PID Tuning"=w242:T9)  [unwired: 3 in]
      n73 = call <vilib>:"PIDController_Pack_AdvTuning.vi"("Filter Derivative"=w263, "MinimumIntegral"=w264, "Kn"=w266, "MaximumIntegral"=w255, "Kf"=w265, "Kd"=w210, "Ki"=w211, "Kp"=w212) -> ("Adv PID Tuning"=w257:T9)  [unwired: 3 in]
      n74 = call <vilib>:"PIDController_Pack_AdvTuning.vi"("Filter Derivative"=w233, "MinimumIntegral"=w234, "Kn"=w236, "MaximumIntegral"=w225, "Kf"=w235, "Kd"=w204, "Ki"=w206, "Kp"=w205) -> ("Adv PID Tuning"=w227:T9)  [unwired: 3 in]
      n75 = call <vilib>:"PIDController_Pack_AdvTuning.vi"("Filter Derivative"=w272, "MinimumIntegral"=w271, "Kn"=w269, "MaximumIntegral"=w280, "Kf"=0.0 ("Kf Arm"), "Kd"=w213, "Ki"=w214, "Kp"=w215) -> ("Adv PID Tuning"=w278:T9)  [unwired: 3 in]
      n76 = call <vilib>:"PIDController_AdvExecute.vi"("Adv PID Limits"=w241, "SP-SetPoint"=170.0 ("Wrist Setpoint"), "PV-Measurement"=w201, "Adv PID Tuning"=w242) -> ("CO-ControlOutput"=w237:dbl)  [unwired: 5 in, 2 out]
      n77 = call <vilib>:"PIDController_AdvExecute.vi"("Time"=w221, "Adv PID Limits"=w256, "SP-SetPoint"=0.0 ("Setpoit Elbow"), "PV-Measurement"=w202, "Adv PID Tuning"=w257) -> ("CO-ControlOutput"=w252:dbl)  [unwired: 4 in, 2 out]
      n78 = call <vilib>:"PIDController_AdvExecute.vi"("Time"=w221, "Adv PID Limits"=w226, "SP-SetPoint"=0.0 ("set point grip"), "PV-Measurement"=w200, "Adv PID Tuning"=w227) -> ("CO-ControlOutput"=w222:dbl)  [unwired: 4 in, 2 out]
      n79 = call <vilib>:"PIDController_AdvExecute.vi"("Time"=w221, "Adv PID Limits"=w279, "SP-SetPoint"=0.0 ("set poit arm"), "PV-Measurement"=w203, "Adv PID Tuning"=w278) -> ("CO-ControlOutput"=w267:dbl)  [unwired: 4 in, 2 out]
    }
    frame "Y" {
      w318 = 1.0  # Kn
      w317 = 0.0  # Kf
      w307 = 9.9e+30  # MaximumIntegral
      w316 = -9.9e+30  # MinimumIntegral
      w315 = FALSE  # Filter Derivative
      w313 = 0.0  # MinInput
      w312 = FALSE  # Continuous
      w311 = 1.0  # MaxOutput
      w314 = -1.0  # MinOutput
      w310 = 1.0  # MaxInput
      w333 = 1.0  # Kn
      w332 = 0.0  # Kf
      w322 = 9.9e+30  # MaximumIntegral
      w331 = -9.9e+30  # MinimumIntegral
      w330 = FALSE  # Filter Derivative
      w328 = 130.0  # MinInput
      w327 = FALSE  # Continuous
      w326 = 1.0  # MaxOutput
      w329 = -1.0  # MinOutput
      w325 = 240.0  # MaxInput
      w348 = 1.0  # Kn
      w347 = 0.0  # Kf
      w337 = 9.9e+30  # MaximumIntegral
      w346 = -9.9e+30  # MinimumIntegral
      w345 = FALSE  # Filter Derivative
      w343 = 0.0  # MinInput
      w342 = FALSE  # Continuous
      w341 = 1.0  # MaxOutput
      w344 = -1.0  # MinOutput
      w340 = 450.0  # MaxInput
      w351 = 1.0  # Kn
      w362 = 9.9e+30  # MaximumIntegral
      w353 = -9.9e+30  # MinimumIntegral
      w354 = FALSE  # Filter Derivative
      w356 = -100.0  # MinInput
      w357 = FALSE  # Continuous
      w358 = 1.0  # MaxOutput
      w355 = -1.0  # MinOutput
      w359 = 100.0  # MaxInput
      # "set point"
      # "BASE"
      # "set point"
      # "set point"
      # "set point"
      # "base postion for movement"
      # "GRAB"
      # "WRIST"
      # "ELBOW"
      # "SHOULDER"
      # "need to change this"
      # "Adv PID\nCtrl"
      # "Adv PID\nCtrl"
      # "Adv PID\nCtrl"
      # "Adv PID\nCtrl"
      n80 = call <vilib>:"Spark MAX Get Absolute Encoder Position.vi"("MotorControlDeviceRef in"=w320) -> ("Position"=w283:dbl)  [unwired: 7 in, 3 out]
      n81 = call <vilib>:"Spark MAX Get Sensor Position.vi"("MotorControlDevRef in"=w335) -> ("Sensor Position"=w284:dbl)  [unwired: 7 in, 3 out]
      n82 = call <vilib>:"Spark MAX Get Sensor Position.vi"("MotorControlDevRef in"=w305) -> ("Sensor Position"=w282:dbl)  [unwired: 7 in, 3 out]
      n83 = call <vilib>:"Spark MAX Get Sensor Position.vi"("MotorControlDevRef in"=w350) -> ("Sensor Position"=w285:dbl)  [unwired: 7 in, 3 out]
      n84 = global read "Robot Global Data.vi" "USB 1 AXIS"() -> (w302:dbl[])
      n85 = Index Array(array=w302, index=XBox_Axes_Indexer."Right X" ("XBox Axes")) -> (element=w300:dbl)
      n86 = call <vilib>:"PIDController_Pack_AdvLimits.vi"("MinOutput"=w329, "MaxOutput"=w326, "Continuous"=w327, "MinInput"=w328, "MaxInput"=w325) -> ("Adv PID Limits"=w323:T8)  [unwired: 6 in]
      n87 = call <vilib>:"PIDController_Pack_AdvLimits.vi"("MinOutput"=w344, "MaxOutput"=w341, "Continuous"=w342, "MinInput"=w343, "MaxInput"=w340) -> ("Adv PID Limits"=w338:T8)  [unwired: 6 in]
      n88 = call <vilib>:"PIDController_Pack_AdvLimits.vi"("MinOutput"=w314, "MaxOutput"=w311, "Continuous"=w312, "MinInput"=w313, "MaxInput"=w310) -> ("Adv PID Limits"=w308:T8)  [unwired: 6 in]
      n89 = call <vilib>:"PIDController_Pack_AdvLimits.vi"("MinOutput"=w355, "MaxOutput"=w358, "Continuous"=w357, "MinInput"=w356, "MaxInput"=w359) -> ("Adv PID Limits"=w361:T8)  [unwired: 6 in]
      n90 = Multiply(x=1.0, y=w300) -> (x*y=w298:dbl)
      n91 = call <vilib>:"PIDController_Pack_AdvTuning.vi"("Filter Derivative"=w330, "MinimumIntegral"=w331, "Kn"=w333, "MaximumIntegral"=w322, "Kf"=w332, "Kd"=w291, "Ki"=w289, "Kp"=w290) -> ("Adv PID Tuning"=w324:T9)  [unwired: 3 in]
      n92 = call <vilib>:"PIDController_Pack_AdvTuning.vi"("Filter Derivative"=w345, "MinimumIntegral"=w346, "Kn"=w348, "MaximumIntegral"=w337, "Kf"=w347, "Kd"=w292, "Ki"=w293, "Kp"=w294) -> ("Adv PID Tuning"=w339:T9)  [unwired: 3 in]
      n93 = call <vilib>:"PIDController_Pack_AdvTuning.vi"("Filter Derivative"=w315, "MinimumIntegral"=w316, "Kn"=w318, "MaximumIntegral"=w307, "Kf"=w317, "Kd"=w286, "Ki"=w288, "Kp"=w287) -> ("Adv PID Tuning"=w309:T9)  [unwired: 3 in]
      n94 = call <vilib>:"PIDController_Pack_AdvTuning.vi"("Filter Derivative"=w354, "MinimumIntegral"=w353, "Kn"=w351, "MaximumIntegral"=w362, "Kf"=0.0 ("Kf Arm"), "Kd"=w295, "Ki"=w296, "Kp"=w297) -> ("Adv PID Tuning"=w360:T9)  [unwired: 3 in]
      n95 = call <vilib>:"PIDController_AdvExecute.vi"("Adv PID Limits"=w323, "SP-SetPoint"=170.0 ("Wrist Setpoint"), "PV-Measurement"=w283, "Adv PID Tuning"=w324) -> ("CO-ControlOutput"=w319:dbl)  [unwired: 5 in, 2 out]
      n96 = call <vilib>:"PIDController_AdvExecute.vi"("Time"=w303, "Adv PID Limits"=w338, "SP-SetPoint"=0.0 ("Setpoit Elbow"), "PV-Measurement"=w284, "Adv PID Tuning"=w339) -> ("CO-ControlOutput"=w334:dbl)  [unwired: 4 in, 2 out]
      n97 = call <vilib>:"PIDController_AdvExecute.vi"("Time"=w303, "Adv PID Limits"=w308, "SP-SetPoint"=0.0 ("set point grip"), "PV-Measurement"=w282, "Adv PID Tuning"=w309) -> ("CO-ControlOutput"=w304:dbl)  [unwired: 4 in, 2 out]
      n98 = call <vilib>:"PIDController_AdvExecute.vi"("Time"=w303, "Adv PID Limits"=w361, "SP-SetPoint"=0.0 ("set poit arm"), "PV-Measurement"=w285, "Adv PID Tuning"=w360) -> ("CO-ControlOutput"=w349:dbl)  [unwired: 4 in, 2 out]
    }
    frame "B" {
      w400 = 1.0  # Kn
      w399 = 0.0  # Kf
      w389 = 9.9e+30  # MaximumIntegral
      w398 = -9.9e+30  # MinimumIntegral
      w397 = FALSE  # Filter Derivative
      w395 = 0.0  # MinInput
      w394 = FALSE  # Continuous
      w393 = 1.0  # MaxOutput
      w396 = -1.0  # MinOutput
      w392 = 1.0  # MaxInput
      w415 = 1.0  # Kn
      w414 = 0.0  # Kf
      w404 = 9.9e+30  # MaximumIntegral
      w413 = -9.9e+30  # MinimumIntegral
      w412 = FALSE  # Filter Derivative
      w410 = 130.0  # MinInput
      w409 = FALSE  # Continuous
      w408 = 1.0  # MaxOutput
      w411 = -1.0  # MinOutput
      w407 = 240.0  # MaxInput
      w430 = 1.0  # Kn
      w429 = 0.0  # Kf
      w419 = 9.9e+30  # MaximumIntegral
      w428 = -9.9e+30  # MinimumIntegral
      w427 = FALSE  # Filter Derivative
      w425 = 0.0  # MinInput
      w424 = FALSE  # Continuous
      w423 = 1.0  # MaxOutput
      w426 = -1.0  # MinOutput
      w422 = 450.0  # MaxInput
      w433 = 1.0  # Kn
      w444 = 9.9e+30  # MaximumIntegral
      w435 = -9.9e+30  # MinimumIntegral
      w436 = FALSE  # Filter Derivative
      w438 = -100.0  # MinInput
      w439 = FALSE  # Continuous
      w440 = 1.0  # MaxOutput
      w437 = -1.0  # MinOutput
      w441 = 100.0  # MaxInput
      # "set point"
      # "BASE"
      # "set point"
      # "set point"
      # "set point"
      # "base postion for movement"
      # "GRAB"
      # "WRIST"
      # "ELBOW"
      # "SHOULDER"
      # "need to change this"
      # "Adv PID\nCtrl"
      # "Adv PID\nCtrl"
      # "Adv PID\nCtrl"
      # "Adv PID\nCtrl"
      n99 = call <vilib>:"Spark MAX Get Absolute Encoder Position.vi"("MotorControlDeviceRef in"=w402) -> ("Position"=w365:dbl)  [unwired: 7 in, 3 out]
      n100 = call <vilib>:"Spark MAX Get Sensor Position.vi"("MotorControlDevRef in"=w417) -> ("Sensor Position"=w366:dbl)  [unwired: 7 in, 3 out]
      n101 = call <vilib>:"Spark MAX Get Sensor Position.vi"("MotorControlDevRef in"=w387) -> ("Sensor Position"=w364:dbl)  [unwired: 7 in, 3 out]
      n102 = call <vilib>:"Spark MAX Get Sensor Position.vi"("MotorControlDevRef in"=w432) -> ("Sensor Position"=w367:dbl)  [unwired: 7 in, 3 out]
      n103 = global read "Robot Global Data.vi" "USB 1 AXIS"() -> (w384:dbl[])
      n104 = Index Array(array=w384, index=XBox_Axes_Indexer."Right X" ("XBox Axes")) -> (element=w382:dbl)
      n105 = call <vilib>:"PIDController_Pack_AdvLimits.vi"("MinOutput"=w411, "MaxOutput"=w408, "Continuous"=w409, "MinInput"=w410, "MaxInput"=w407) -> ("Adv PID Limits"=w405:T8)  [unwired: 6 in]
      n106 = call <vilib>:"PIDController_Pack_AdvLimits.vi"("MinOutput"=w426, "MaxOutput"=w423, "Continuous"=w424, "MinInput"=w425, "MaxInput"=w422) -> ("Adv PID Limits"=w420:T8)  [unwired: 6 in]
      n107 = call <vilib>:"PIDController_Pack_AdvLimits.vi"("MinOutput"=w396, "MaxOutput"=w393, "Continuous"=w394, "MinInput"=w395, "MaxInput"=w392) -> ("Adv PID Limits"=w390:T8)  [unwired: 6 in]
      n108 = call <vilib>:"PIDController_Pack_AdvLimits.vi"("MinOutput"=w437, "MaxOutput"=w440, "Continuous"=w439, "MinInput"=w438, "MaxInput"=w441) -> ("Adv PID Limits"=w443:T8)  [unwired: 6 in]
      n109 = Multiply(x=1.0, y=w382) -> (x*y=w380:dbl)
      n110 = call <vilib>:"PIDController_Pack_AdvTuning.vi"("Filter Derivative"=w412, "MinimumIntegral"=w413, "Kn"=w415, "MaximumIntegral"=w404, "Kf"=w414, "Kd"=w373, "Ki"=w371, "Kp"=w372) -> ("Adv PID Tuning"=w406:T9)  [unwired: 3 in]
      n111 = call <vilib>:"PIDController_Pack_AdvTuning.vi"("Filter Derivative"=w427, "MinimumIntegral"=w428, "Kn"=w430, "MaximumIntegral"=w419, "Kf"=w429, "Kd"=w374, "Ki"=w375, "Kp"=w376) -> ("Adv PID Tuning"=w421:T9)  [unwired: 3 in]
      n112 = call <vilib>:"PIDController_Pack_AdvTuning.vi"("Filter Derivative"=w397, "MinimumIntegral"=w398, "Kn"=w400, "MaximumIntegral"=w389, "Kf"=w399, "Kd"=w368, "Ki"=w370, "Kp"=w369) -> ("Adv PID Tuning"=w391:T9)  [unwired: 3 in]
      n113 = call <vilib>:"PIDController_Pack_AdvTuning.vi"("Filter Derivative"=w436, "MinimumIntegral"=w435, "Kn"=w433, "MaximumIntegral"=w444, "Kf"=0.0 ("Kf Arm"), "Kd"=w377, "Ki"=w378, "Kp"=w379) -> ("Adv PID Tuning"=w442:T9)  [unwired: 3 in]
      n114 = call <vilib>:"PIDController_AdvExecute.vi"("Adv PID Limits"=w405, "SP-SetPoint"=170.0 ("Wrist Setpoint"), "PV-Measurement"=w365, "Adv PID Tuning"=w406) -> ("CO-ControlOutput"=w401:dbl)  [unwired: 5 in, 2 out]
      n115 = call <vilib>:"PIDController_AdvExecute.vi"("Time"=w385, "Adv PID Limits"=w420, "SP-SetPoint"=0.0 ("Setpoit Elbow"), "PV-Measurement"=w366, "Adv PID Tuning"=w421) -> ("CO-ControlOutput"=w416:dbl)  [unwired: 4 in, 2 out]
      n116 = call <vilib>:"PIDController_AdvExecute.vi"("Time"=w385, "Adv PID Limits"=w390, "SP-SetPoint"=0.0 ("set point grip"), "PV-Measurement"=w364, "Adv PID Tuning"=w391) -> ("CO-ControlOutput"=w386:dbl)  [unwired: 4 in, 2 out]
      n117 = call <vilib>:"PIDController_AdvExecute.vi"("Time"=w385, "Adv PID Limits"=w443, "SP-SetPoint"=0.0 ("set poit arm"), "PV-Measurement"=w367, "Adv PID Tuning"=w442) -> ("CO-ControlOutput"=w431:dbl)  [unwired: 4 in, 2 out]
    }
    frame "A" {
      w482 = 1.0  # Kn
      w481 = 0.0  # Kf
      w471 = 9.9e+30  # MaximumIntegral
      w480 = -9.9e+30  # MinimumIntegral
      w479 = FALSE  # Filter Derivative
      w477 = 0.0  # MinInput
      w476 = FALSE  # Continuous
      w475 = 1.0  # MaxOutput
      w478 = -1.0  # MinOutput
      w474 = 1.0  # MaxInput
      w497 = 1.0  # Kn
      w496 = 0.0  # Kf
      w486 = 9.9e+30  # MaximumIntegral
      w495 = -9.9e+30  # MinimumIntegral
      w494 = FALSE  # Filter Derivative
      w492 = 130.0  # MinInput
      w491 = FALSE  # Continuous
      w490 = 1.0  # MaxOutput
      w493 = -1.0  # MinOutput
      w489 = 240.0  # MaxInput
      w512 = 1.0  # Kn
      w511 = 0.0  # Kf
      w501 = 9.9e+30  # MaximumIntegral
      w510 = -9.9e+30  # MinimumIntegral
      w509 = FALSE  # Filter Derivative
      w507 = 0.0  # MinInput
      w506 = FALSE  # Continuous
      w505 = 1.0  # MaxOutput
      w508 = -1.0  # MinOutput
      w504 = 450.0  # MaxInput
      w515 = 1.0  # Kn
      w526 = 9.9e+30  # MaximumIntegral
      w517 = -9.9e+30  # MinimumIntegral
      w518 = FALSE  # Filter Derivative
      w520 = -100.0  # MinInput
      w521 = FALSE  # Continuous
      w522 = 1.0  # MaxOutput
      w519 = -1.0  # MinOutput
      w523 = 100.0  # MaxInput
      # "set point"
      # "BASE"
      # "set point"
      # "set point"
      # "set point"
      # "base postion for movement"
      # "GRAB"
      # "WRIST"
      # "ELBOW"
      # "SHOULDER"
      # "need to change this"
      # "Adv PID\nCtrl"
      # "Adv PID\nCtrl"
      # "Adv PID\nCtrl"
      # "Adv PID\nCtrl"
      n118 = call <vilib>:"Spark MAX Get Absolute Encoder Position.vi"("MotorControlDeviceRef in"=w484) -> ("Position"=w447:dbl)  [unwired: 7 in, 3 out]
      n119 = call <vilib>:"Spark MAX Get Sensor Position.vi"("MotorControlDevRef in"=w499) -> ("Sensor Position"=w448:dbl)  [unwired: 7 in, 3 out]
      n120 = call <vilib>:"Spark MAX Get Sensor Position.vi"("MotorControlDevRef in"=w469) -> ("Sensor Position"=w446:dbl)  [unwired: 7 in, 3 out]
      n121 = call <vilib>:"Spark MAX Get Sensor Position.vi"("MotorControlDevRef in"=w514) -> ("Sensor Position"=w449:dbl)  [unwired: 7 in, 3 out]
      n122 = global read "Robot Global Data.vi" "USB 1 AXIS"() -> (w466:dbl[])
      n123 = Index Array(array=w466, index=XBox_Axes_Indexer."Right X" ("XBox Axes")) -> (element=w464:dbl)
      n124 = call <vilib>:"PIDController_Pack_AdvLimits.vi"("MinOutput"=w493, "MaxOutput"=w490, "Continuous"=w491, "MinInput"=w492, "MaxInput"=w489) -> ("Adv PID Limits"=w487:T8)  [unwired: 6 in]
      n125 = call <vilib>:"PIDController_Pack_AdvLimits.vi"("MinOutput"=w508, "MaxOutput"=w505, "Continuous"=w506, "MinInput"=w507, "MaxInput"=w504) -> ("Adv PID Limits"=w502:T8)  [unwired: 6 in]
      n126 = call <vilib>:"PIDController_Pack_AdvLimits.vi"("MinOutput"=w478, "MaxOutput"=w475, "Continuous"=w476, "MinInput"=w477, "MaxInput"=w474) -> ("Adv PID Limits"=w472:T8)  [unwired: 6 in]
      n127 = call <vilib>:"PIDController_Pack_AdvLimits.vi"("MinOutput"=w519, "MaxOutput"=w522, "Continuous"=w521, "MinInput"=w520, "MaxInput"=w523) -> ("Adv PID Limits"=w525:T8)  [unwired: 6 in]
      n128 = Multiply(x=1.0, y=w464) -> (x*y=w462:dbl)
      n129 = call <vilib>:"PIDController_Pack_AdvTuning.vi"("Filter Derivative"=w494, "MinimumIntegral"=w495, "Kn"=w497, "MaximumIntegral"=w486, "Kf"=w496, "Kd"=w455, "Ki"=w453, "Kp"=w454) -> ("Adv PID Tuning"=w488:T9)  [unwired: 3 in]
      n130 = call <vilib>:"PIDController_Pack_AdvTuning.vi"("Filter Derivative"=w509, "MinimumIntegral"=w510, "Kn"=w512, "MaximumIntegral"=w501, "Kf"=w511, "Kd"=w456, "Ki"=w457, "Kp"=w458) -> ("Adv PID Tuning"=w503:T9)  [unwired: 3 in]
      n131 = call <vilib>:"PIDController_Pack_AdvTuning.vi"("Filter Derivative"=w479, "MinimumIntegral"=w480, "Kn"=w482, "MaximumIntegral"=w471, "Kf"=w481, "Kd"=w450, "Ki"=w452, "Kp"=w451) -> ("Adv PID Tuning"=w473:T9)  [unwired: 3 in]
      n132 = call <vilib>:"PIDController_Pack_AdvTuning.vi"("Filter Derivative"=w518, "MinimumIntegral"=w517, "Kn"=w515, "MaximumIntegral"=w526, "Kf"=0.0 ("Kf Arm"), "Kd"=w459, "Ki"=w460, "Kp"=w461) -> ("Adv PID Tuning"=w524:T9)  [unwired: 3 in]
      n133 = call <vilib>:"PIDController_AdvExecute.vi"("Adv PID Limits"=w487, "SP-SetPoint"=170.0 ("Wrist Setpoint"), "PV-Measurement"=w447, "Adv PID Tuning"=w488) -> ("CO-ControlOutput"=w483:dbl)  [unwired: 5 in, 2 out]
      n134 = call <vilib>:"PIDController_AdvExecute.vi"("Time"=w467, "Adv PID Limits"=w502, "SP-SetPoint"=0.0 ("Setpoit Elbow"), "PV-Measurement"=w448, "Adv PID Tuning"=w503) -> ("CO-ControlOutput"=w498:dbl)  [unwired: 4 in, 2 out]
      n135 = call <vilib>:"PIDController_AdvExecute.vi"("Time"=w467, "Adv PID Limits"=w472, "SP-SetPoint"=0.0 ("set point grip"), "PV-Measurement"=w446, "Adv PID Tuning"=w473) -> ("CO-ControlOutput"=w468:dbl)  [unwired: 4 in, 2 out]
      n136 = call <vilib>:"PIDController_AdvExecute.vi"("Time"=w467, "Adv PID Limits"=w525, "SP-SetPoint"=0.0 ("set poit arm"), "PV-Measurement"=w449, "Adv PID Tuning"=w524) -> ("CO-ControlOutput"=w513:dbl)  [unwired: 4 in, 2 out]
    }
  }
  "current angle" <- w4
  "current angle 2" <- w3
  "current angle 3" <- w2
  "current angle 5" <- w1
  n137 = Build Array(w38, w37, w36, w35, w34) -> (→"appended array 2":dbl[])
